vi "Magazine_Teleop.vi"(11 "Joystick_Out":T1) -> ()   [LabVIEW 2019]
uses:
  Utility VIs/Joystick_Controls.ctl
  Subsystems/Magazine/Magazine_Cluster.ctl
  Subsystems/Magazine/Magazine_States.ctl
  Globals/Magazine_Globals.vi
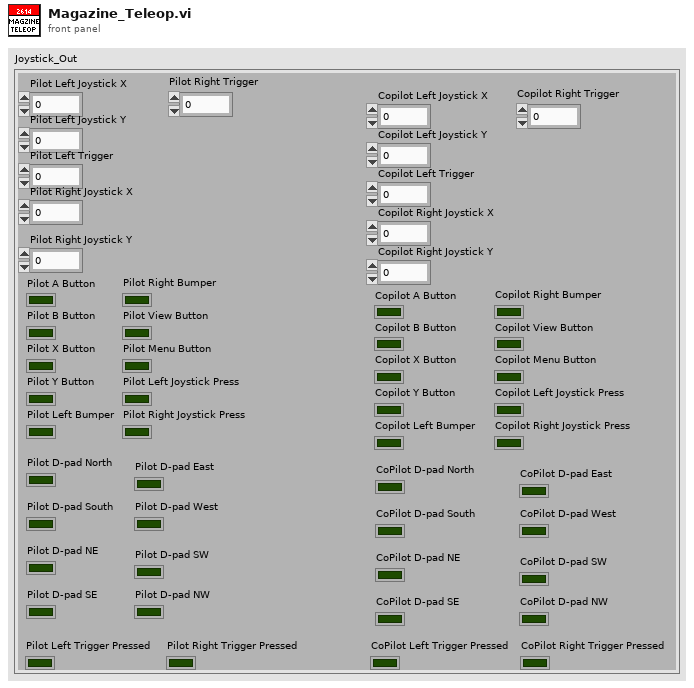
[diagram p1: front panel]
types:
  T1 = typedef "Joystick_Controls.ctl" = cluster{"Pilot Left Joystick X":dbl, "Pilot Left Joystick Y":dbl, "Pilot A Button":bool, "Pilot B Button":bool, "Pilot X Button":bool, "Pilot Y Button":bool, "Pilot Left Bumper":bool, "Pilot Right Bumper":bool, "Pilot View Button":bool, "Pilot Menu Button":bool, "Pilot Left Joystick Press":bool, "Pilot Right Joystick Press":bool, "Pilot Left Trigger":dbl, "Pilot Right Joystick X":dbl, "Pilot Right Joystick Y":dbl, "Pilot Right Trigger":dbl, "Copilot Left Joystick X":dbl, "Copilot Left Joystick Y":dbl, "Copilot A Button":bool, "Copilot B Button":bool, "Copilot X Button":bool, "Copilot Y Button":bool, "Copilot Left Bumper":bool, "Copilot Right Bumper":bool, "Copilot View Button":bool, "Copilot Menu Button":bool, "Copilot Left Joystick Press":bool, "Copilot Right Joystick Press":bool, "Copilot Left Trigger":dbl, "Copilot Right Joystick X":dbl, "Copilot Right Joystick Y":dbl, "Copilot Right Trigger":dbl, "Pilot D-pad North":bool, "Pilot D-pad South":bool, "Pilot D-pad East":bool, "Pilot D-pad West":bool, "Pilot D-pad NE ":bool, "Pilot D-pad SE":bool, "Pilot D-pad SW":bool, "Pilot D-pad NW":bool, "CoPilot D-pad North":bool, "CoPilot D-pad South":bool, "CoPilot D-pad East":bool, "CoPilot D-pad West":bool, "CoPilot D-pad NE":bool, "CoPilot D-pad SE":bool, "CoPilot D-pad SW":bool, "CoPilot D-pad NW":bool, "Pilot Left Trigger Pressed":bool, "Pilot Right Trigger Pressed":bool, "CoPilot Left Trigger Pressed":bool, "CoPilot Right Trigger Pressed":bool}
  T2 = typedef "Magazine_Cluster.ctl" = cluster{"Control_States":T3, "Magazine_Throttle":dbl, "Firing":bool}
  T3 = typedef "Magazine_States.ctl" = enum16{"No-Op", "Manual_%Vbus", "Firing", ""}
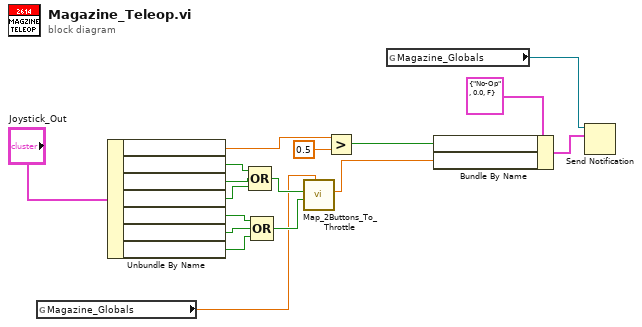
[diagram p0: block diagram]
diagram:
  n1 = global read "Magazine_Globals.vi" item#8() -> (w1:dbl)
  n2 = Unbundle By Name("Joystick_Out") -> (w4:dbl, w13:bool, w12:bool, w11:bool, w10:bool, w9:bool, w8:bool)
  n3 = Compound Arithmetic op=OR(w13, w12, w11) -> (w7:bool)
  n4 = Compound Arithmetic op=OR(w10, w9, w8) -> (w6:bool)
  n5 = call "Map_2Buttons_To_Throttle.vi"(7:w1, 9:w6, 10:w7) -> (2:w5:dbl)  [unwired: 8 in]
  n6 = Greater?(x=w4, y=0.5) -> (0:w2:bool)
  n7 = global read "Magazine_Globals.vi" item#2() -> (w15:refnum<notifier>)
  n8 = Bundle By Name(cluster=T2 {"Control_States"=enum."No-Op", "Magazine_Throttle"=0.0, "Firing"=FALSE} ("Cluster"), w2, w5) -> (w14:T2)
  n9 = Send Notification(notification=w14, notifier=w15) -> ()  [unwired: 1 in, 2 out]
